vi "读取数据发送次数.vi"(8 "error in (no error)":errorcluster caption="错误输入（无错误）", 11 "data_combination输入":refnum<class "data_combination.lvclass">) -> (0 "error out":errorcluster caption="错误输出", 2 "数据发送次数":i32, 3 "data_combination输出":refnum<class "data_combination.lvclass">)   [LabVIEW 2016, in "中水三立SQL数据传输.lvlib" / "data_combination.lvclass"]
uses:
  data_combination.lvclass
  data_combination.lvclass/data_combination.ctl
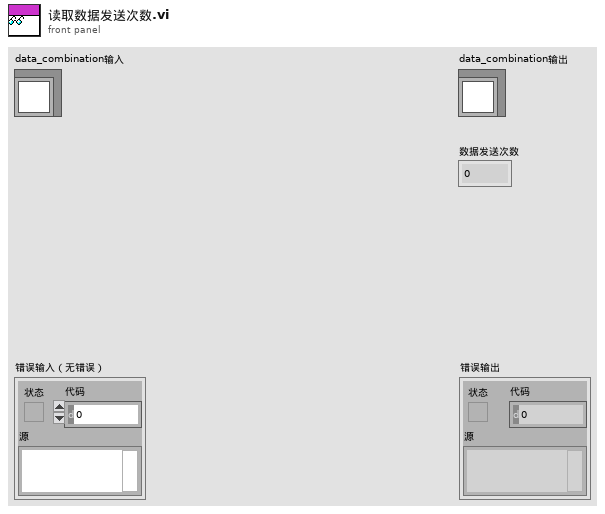
[diagram p1: front panel]
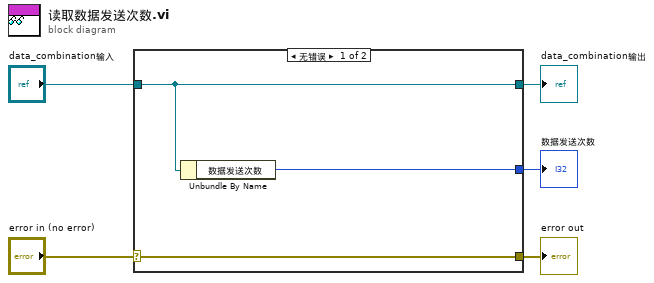
[diagram p0: block diagram]
diagram:
  n1 = case shown="无错误" "error in (no error)" {
    selector: "error in (no error)" -> [w8 w9]
    tunnel: [w8 w9] -> w4
    tunnel: [w7 w10] -> w2
    tunnel: "data_combination输入" -> [w7 w10]
    tunnel: [w6 _] -> w1
    frame No Error {
      n2 = Unbundle By Name(w7) -> ("数据发送次数"=w6:i32)
    }
    frame Error {
    }
  }
  "error out" <- w4
  "data_combination输出" <- w2
  "数据发送次数" <- w1
